vi "Async Logger.vi"(8 "error in":errorcluster, 11 "Logger Parameters":T1) -> (0 "error out":errorcluster, 3 "Logger Parameters":T1={"State"=enum."Initialize", "is Shutdown"=FALSE, "FIFO Refs"={"All System Channels Data"=refnum, "Status"=refnum, "CPU-RAM Data"=refnum}, "Buffers"={"Size"=0, "Current Index"=0, "Array Size"=0, "All System Channels Data"=[], "LOG Data"=[], "CPU-RAM Data"=[], "CPU-RAM Array"=[]}, "Log File"={"Path"=path "C:/logs/AdvancedTDMS_Telemetry_Prototype.tdms", "Ref"=refnum, "Overwrite File If Exists?"=FALSE, "System Channels"={"Names"=[], "Properties"=[], "Telemetry System Path"=""}}, "Target Info"={"Target Rate (Hz)"=0.0, "# of CPUs"=0, "TotalPhysMem (KB)"=0.0}, "Expected Channels"={"Names"=[], "Indexes"=[], "Count"=0}})   [LabVIEW 2019, in "Telemetry Engine.lvlib"]
uses:
  Telemetry Engine.lvlib
  Types/Logger Data.ctl
  Types/Async Logger State Data.ctl
  Types/System Channels.ctl
  Types/Target Info.ctl
  <vilib>/Platform/TimedLoop/XDataNode/timing_clust.ctl
  <vilib>/Platform/TimedLoop/XDataNode/nitl_modes.ctl
  <vilib>/Platform/TimedLoop/XDataNode/wakeup.ctl
  <vilib>/nisyscfg/Close (System).vi
  <vilib>/platform/TimedLoop/XDataNode/XDataNode.xnode
  <vilib>/Platform/TimedLoop/XDataNode/XDNodeRunTimeDep.lvlib
  <resource>/objmgr/nisysapi.rc
  <vilib>/nisyscfg/nisyscfg.lvlib
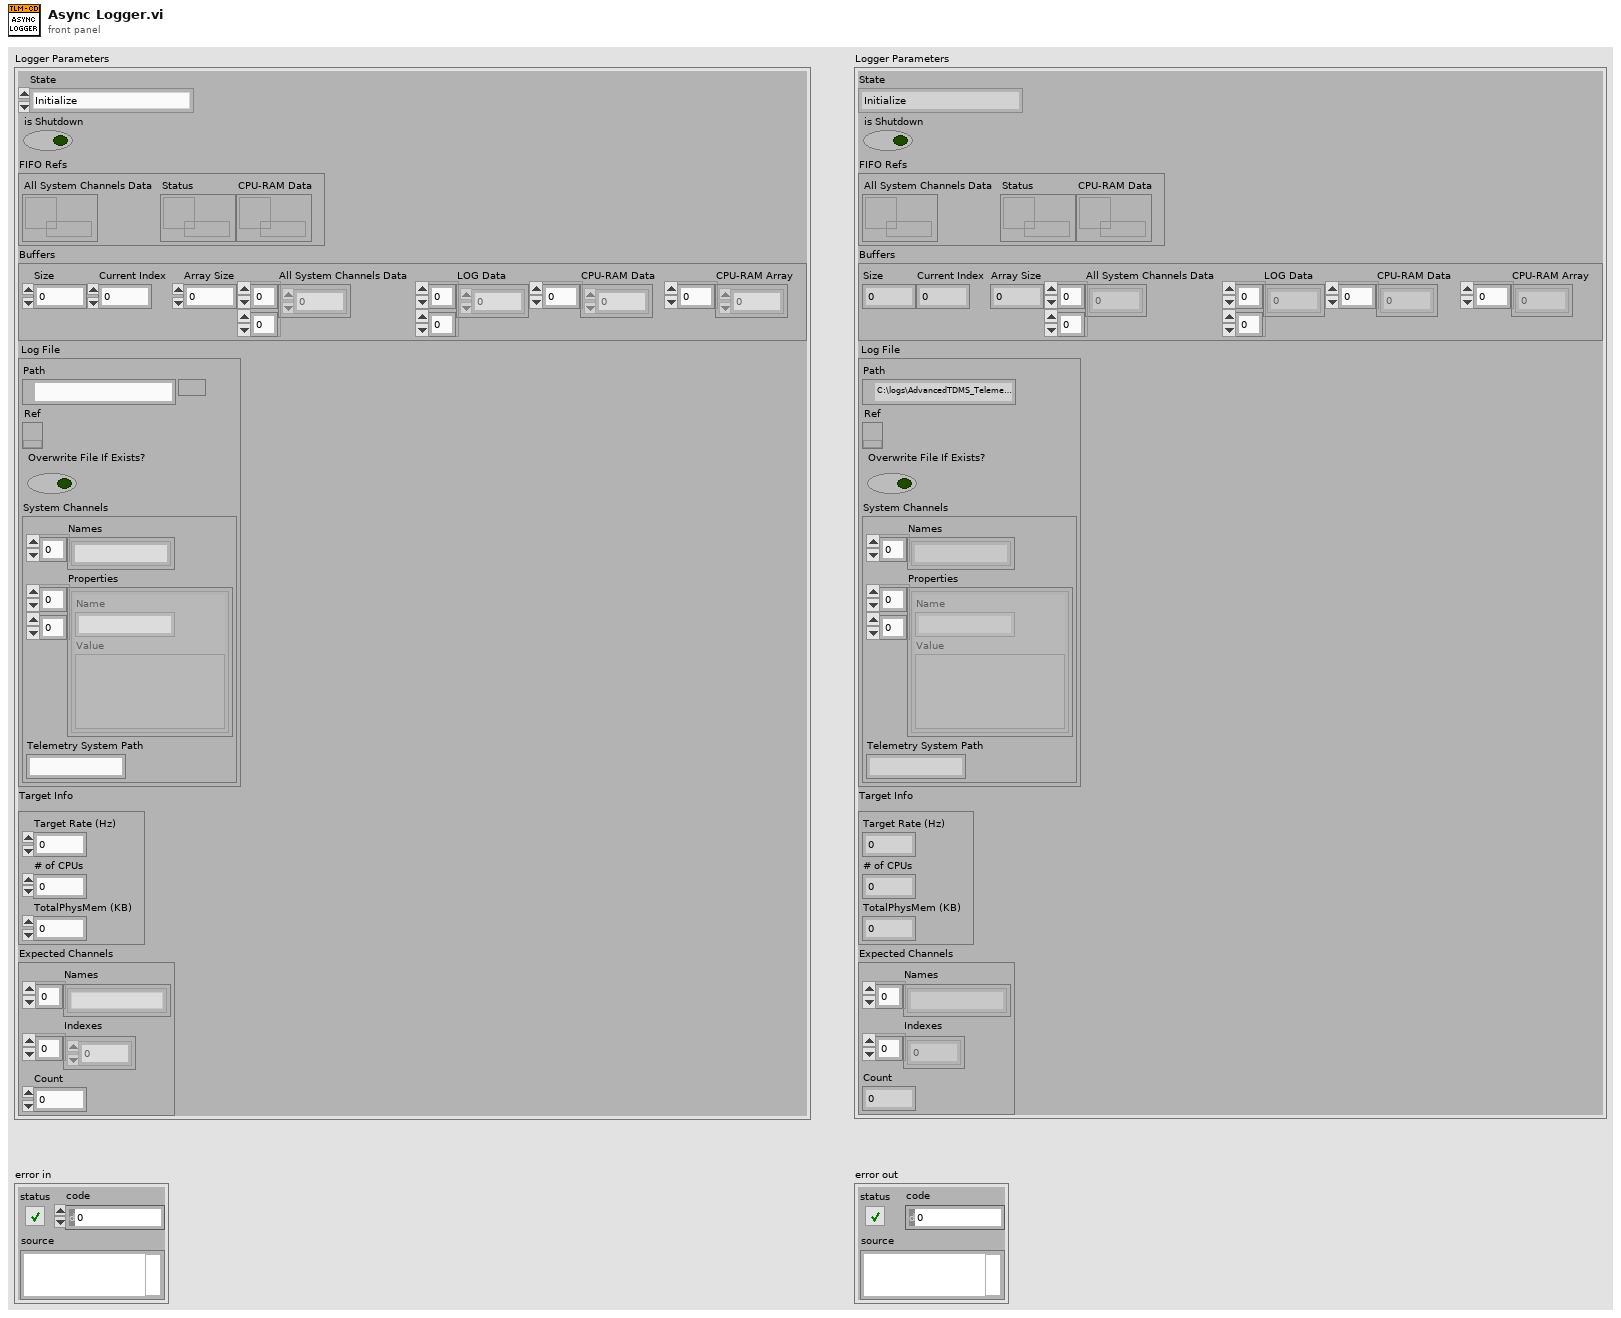
[diagram p1: front panel]
types:
  T1 = typedef "Telemetry Engine.lvlib/Logger Data.ctl" = cluster{"State":T2, "is Shutdown":bool, "FIFO Refs":cluster{"All System Channels Data":refnum<k33>, "Status":refnum<k33>, "CPU-RAM Data":refnum<k33>}, "Buffers":cluster{"Size":i32, "Current Index":i32, "Array Size":i32, "All System Channels Data":dbl[][], "LOG Data":dbl[][], "CPU-RAM Data":dbl[], "CPU-RAM Array":dbl[]}, "Log File":cluster{"Path":path, "Ref":refnum<k34>, "Overwrite File If Exists?":bool, "System Channels":T3}, "Target Info":T4, "Expected Channels":cluster{"Names":string[], "Indexes":i32[], "Count":i32}}
  T2 = typedef "Telemetry Engine.lvlib/Async Logger State Data.ctl" = enum16{"Initialize", "Read System Channels FIFO", "Filter System Channels", "Read CPU-RAM FIFO", "Log Data", "Shutdown"}
  T3 = typedef "Telemetry Engine.lvlib/System Channels.ctl" = cluster{"Names":string[], "Properties":cluster{"Name":string, "Value":variant}[][], "Telemetry System Path":string}
  T4 = typedef "Telemetry Engine.lvlib/Target Info.ctl" = cluster{"Target Rate (Hz)":dbl, "# of CPUs":u32, "TotalPhysMem (KB)":dbl}
  T5 = typedef "XDNodeRunTimeDep.lvlib/timing_clust.ctl" = cluster{"Expected End [f-1]":u64, "Actual End [f-1]":u64, "Finished Late? [f-1]":bool, "Expected End [i-1]":u64, "Actual End [i-1]":u64, "Finished Late? [i-1]":bool, "Expected Start [i]":u64, "Actual Start [i]":u64, "Expected Start [f]":u64, "Actual Start [f]":u64, "Source Name":string, "Structure Name":string, "Period":i64, "Deadline":i64, "Offset":i64, "Start":i64, "Priority":i32, "Timeout":i32, "Mode":T6, "Wakeup Reason":T7, "Error":errorcluster, "Source Type":string, "Secondary Source Type":string, "Global End Time":u64, "Global Start Time":u64, "Frame Duration":u64, "Iteration Duration":u64, "Assigned CPU":i32, "I/O Scan Engine Mode":u32}
  T6 = typedef "XDNodeRunTimeDep.lvlib/nitl_modes.ctl" = enum32{"No Change", "Process missed periods, maintain original phase", "Discard missed periods, maintain original phase", "Process missed periods, ignore original phase", "Discard missed periods, ignore original phase"}
  T7 = typedef "XDNodeRunTimeDep.lvlib/wakeup.ctl" = enum32{"Normal", "Aborted", "Asynchronous wakeup", "Timing source error", "Timed loop error", "Timeout"}
  T8 = typedef "NI_Real-Time Target Support.lvlib/RT CPU Load.ctl" = cluster{"Total (%)":dbl, "Time Critical (%)":dbl, "Timed Structures (%)":dbl, "High (%)":dbl, "Above Normal (%)":dbl, "Normal (%)":dbl, "Background (%)":dbl, "Idle (%)":dbl, "ISR (%)":dbl}
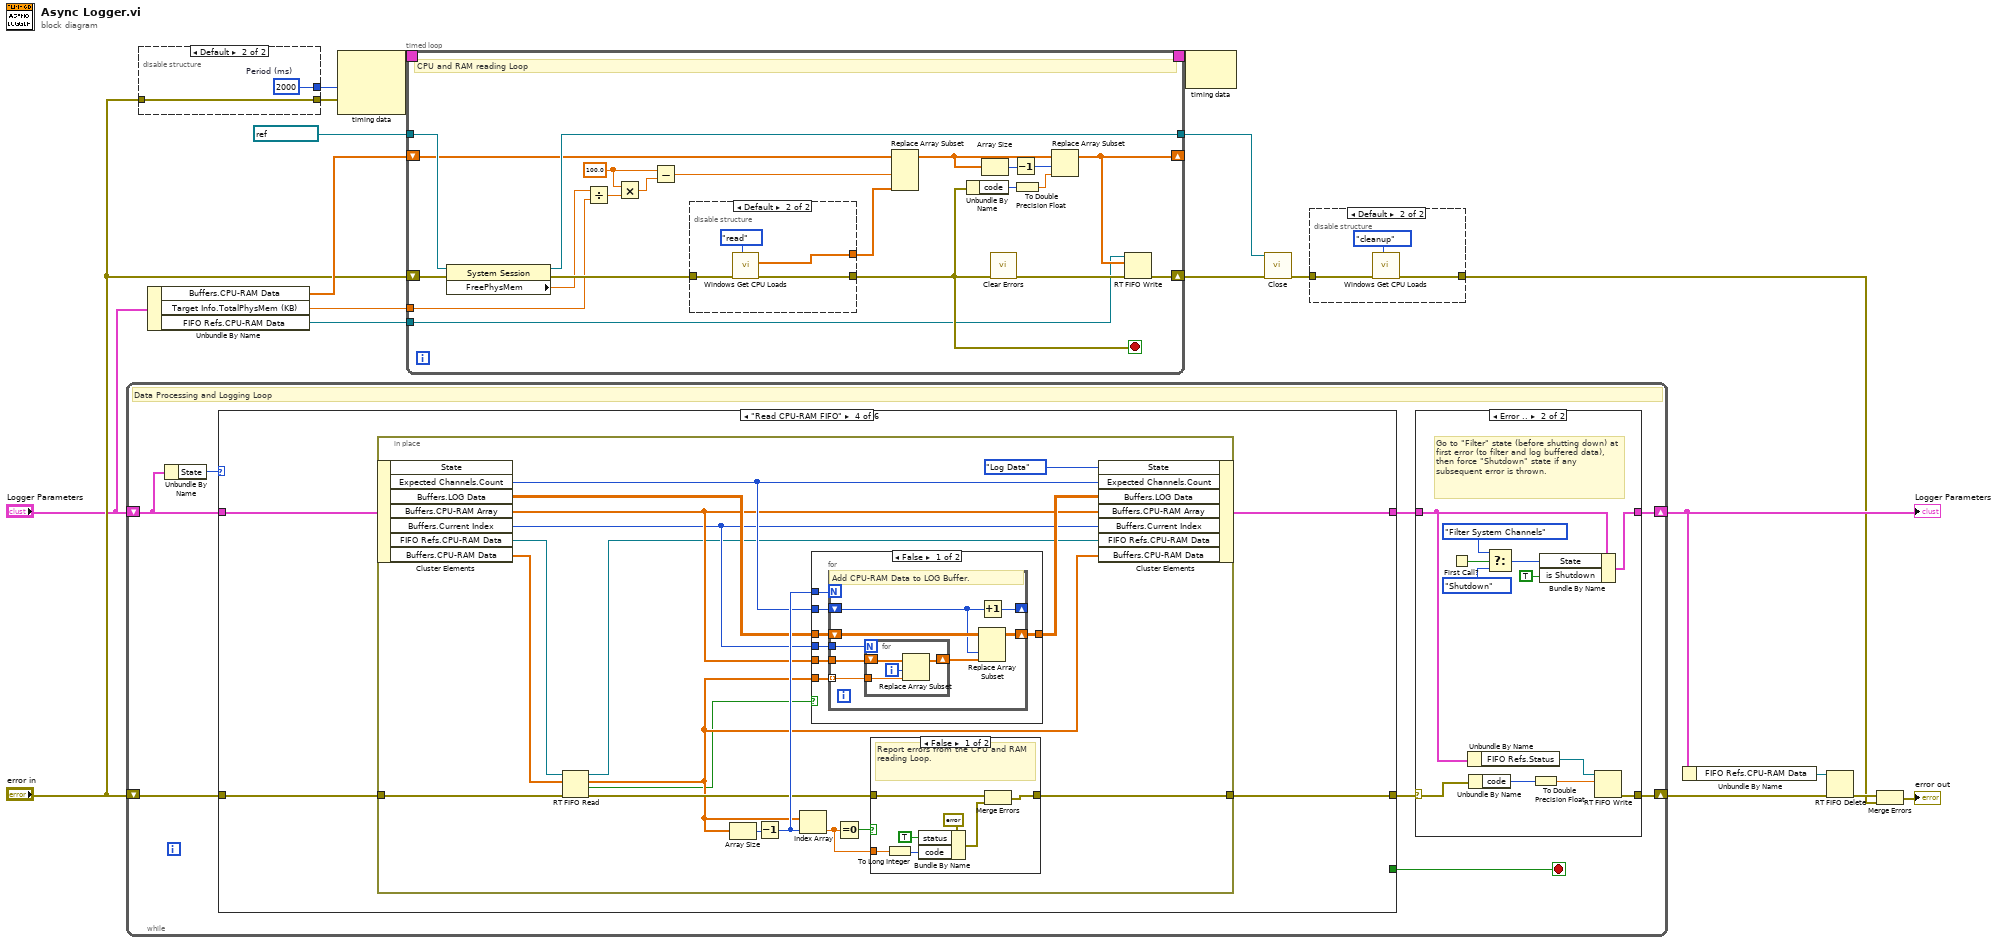
[diagram p0: block diagram]
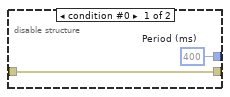
[diagram p3: hidden frame]
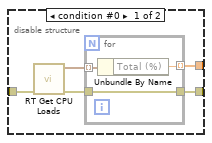
[diagram p4: hidden frame]
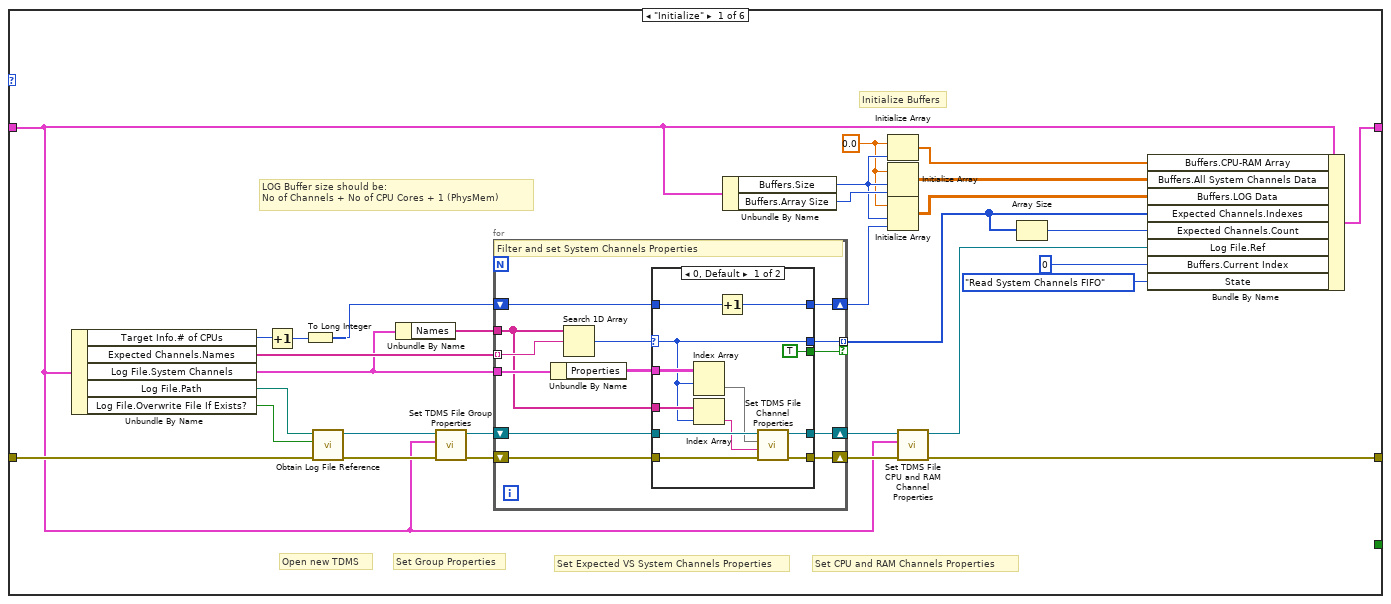
[diagram p5: hidden frame]
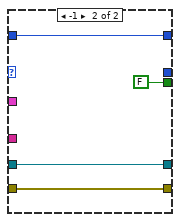
[diagram p6: hidden frame]
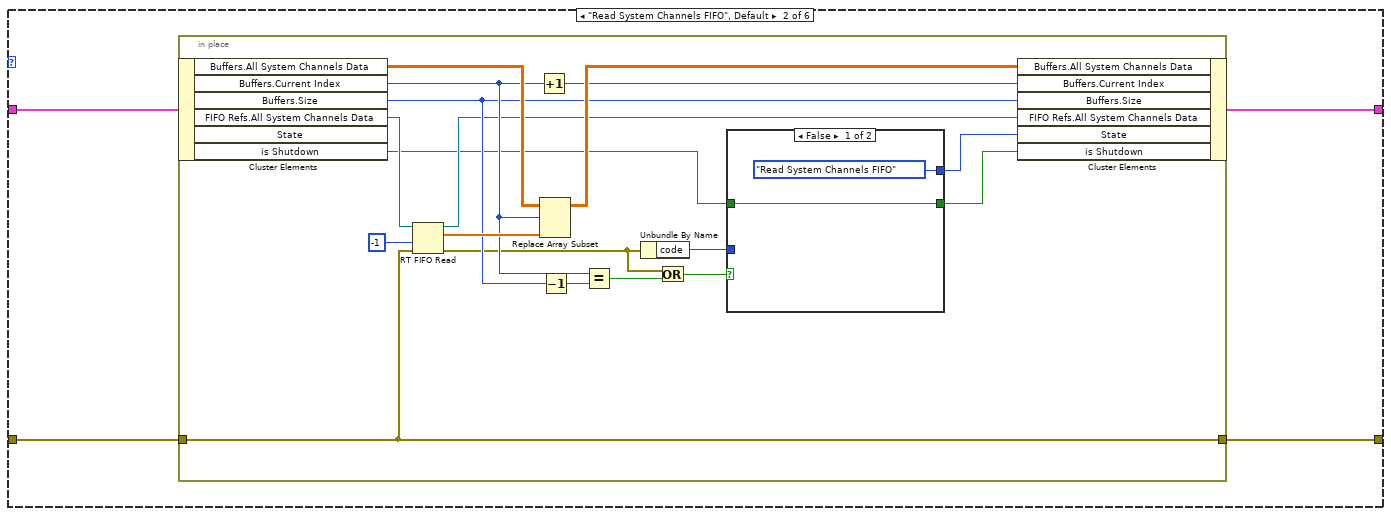
[diagram p7: hidden frame]
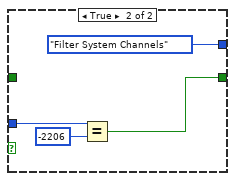
[diagram p8: hidden frame]
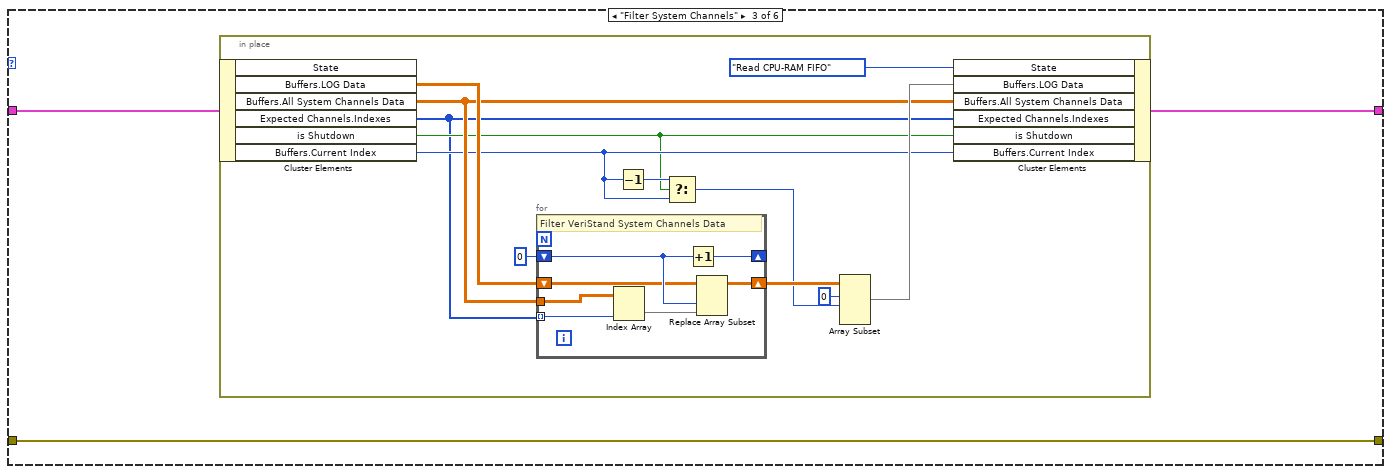
[diagram p9: hidden frame]
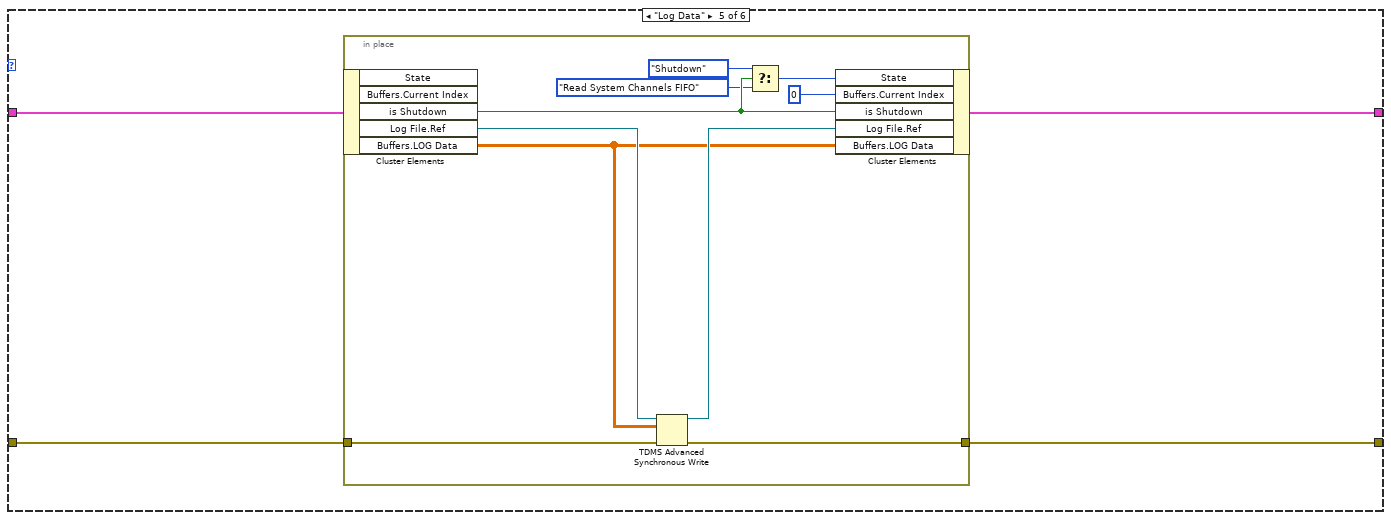
[diagram p12: hidden frame]
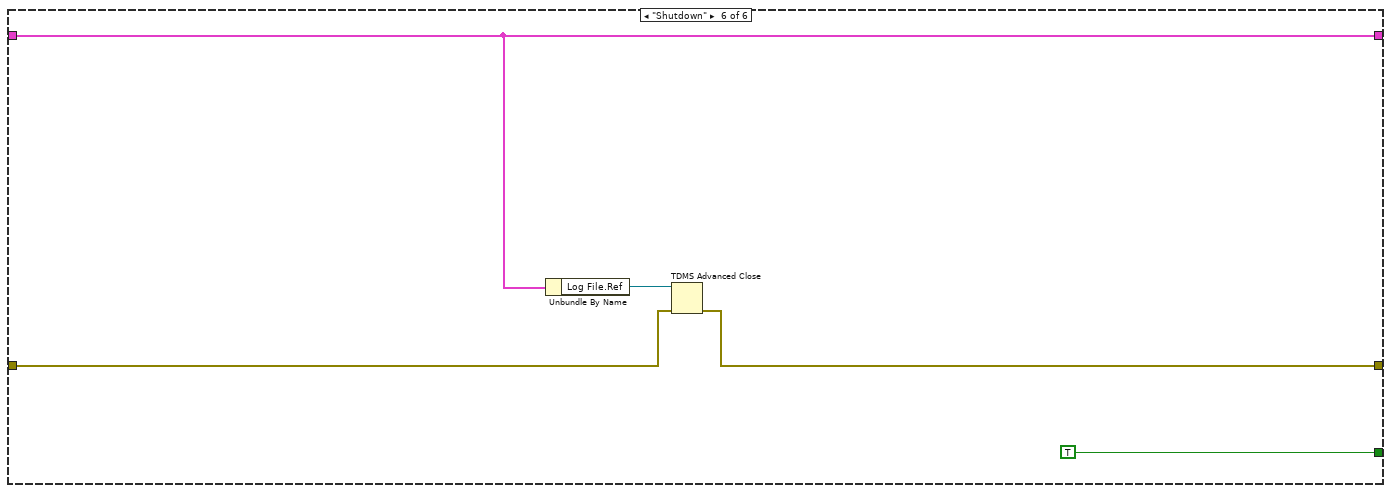
[diagram p13: hidden frame]
diagram:
  n1 = while {
    shift-right: [w22] -> w12
    shift-left: "Logger Parameters" -> [w21]
    shift-right: [w25] -> w14
    shift-left: "error in" -> [w26]
    stop <- w27 stop-if-true
    # "Data Processing and Logging Loop"
    n2 = Unbundle By Name(w21) -> ("State"=w20:T2)
    n3 = case shown="\"Read CPU-RAM FIFO\"" w20 {
      tunnel: [_ _ _ _ _ TRUE] -> w27
      tunnel: w21 -> [w28 w87 w117 w140 w188 w204]
      tunnel: [w55 w90 w116 w139 w187 w204] -> w23
      tunnel: [w37 w88 w115 w137 w189 w201] -> w24
      tunnel: w26 -> [w50 w89 w115 w138 w190 w202]
      frame "Initialize" {
        w29 = 0.0 ("element")
        # "Initialize Buffers"
        # "Set CPU and RAM Channels Properties"
        # "Set Expected VS System Channels Properties"
        # "Set Group Properties"
        # "Open new TDMS"
        # "LOG Buffer size should be:\nNo of Channels + No of CPU Cores + 1 (PhysMem)"
        n4 = Unbundle By Name(w28) -> ("Target Info.# of CPUs"=w41:u32, "Expected Channels.Names"=w47:string[], "Log File.System Channels"=w42:T3, "Log File.Path"=w49:path, "Log File.Overwrite File If Exists?"=w51:bool)
        n5 = Increment(x=w41) -> (x+1=w40:u32)
        n6 = To Long Integer(number=w40) -> (32bit integer=w39:i32)
        n7 = call "Obtain Log File Reference.vi"("error in"=w50, "Overwrite File If Exists?"=w51, "Log File Path"=w49) -> ("error out"=w45:errorcluster, "Log File Refnum out"=w43:refnum<k34>)  [unwired: 7 in]
        n8 = Unbundle By Name(w42) -> ("Names"=w48:string[])
        n9 = call "Set TDMS File Group Properties.vi"("error in (no error)"=w45, "Logger Parameters"=w28, "Refnum in"=w43) -> ("error out"=w46:errorcluster, "Refnum out"=w44:refnum<k34>)  [unwired: 7 in]
        n10 = for {
          shift-right: [w68] -> w36
          shift-left: w44 -> [w69]
          shift-right: [w67] -> w38
          shift-left: w46 -> [w70]
          shift-right: [w65] -> w54
          shift-left: w39 -> [w66]
          tunnel: w47 -> [w63] mode=indexing
          tunnel: w48 -> [w58]
          tunnel: [w62] -> w33 mode=indexing if=w59
          tunnel: w42 -> [w61]
          # "Filter and set System Channels Properties"
          n11 = Unbundle By Name(w61) -> ("Properties"=w60:cluster{"Name":string, "Value":variant}[][])
          n12 = Search 1D Array(1D array=w58, element=w63) -> (index of element=w64:i32)  [unwired: 1 in]
          n13 = case shown="0, Default" w64 {
            selector: w64 -> [w72 _]
            tunnel: [w82 w86] -> w68
            tunnel: [w81 w84] -> w67
            tunnel: w70 -> [w80 w84]
            tunnel: w69 -> [w79 w86]
            tunnel: w66 -> [w78 w85]
            tunnel: [w77 w85] -> w65
            tunnel: [w72 _] -> w62
            tunnel: w60 -> [w76 _]
            tunnel: [TRUE FALSE] -> w59
            tunnel: w58 -> [w73 _]
            frame 0, Default {
              n14 = Index Array(array=w76, index (row)=w72) -> (element=w75:cluster{"Name":string, "Value":variant}[])  [unwired: 1 in]
              n15 = Index Array(array=w73, index=w72) -> (element=w71:string)
              n16 = Increment(x=w78) -> (x+1=w77:i32)
              n17 = call "Set TDMS File Channel Properties.vi"("error in (no error)"=w80, "Channel Name"=w71, "Channel Properties"=w75, "tdms file in"=w79) -> ("error out"=w81:errorcluster, "tdms file out"=w82:refnum<k34>)  [unwired: 6 in]
            }
            frame -1 {
            }
          }
        }
        n18 = Unbundle By Name(w28) -> ("Buffers.Size"=w30:i32, "Buffers.Array Size"=w57:i32)
        n19 = Initialize Array(w29, w30) -> (w31:dbl[])
        n20 = Initialize Array(w29, w30, w57) -> (w56:dbl[][])
        n21 = Initialize Array(w29, w30, w54) -> (w53:dbl[][])
        n22 = call "Set TDMS File CPU and RAM Channel Properties.vi"("error in (no error)"=w38, "Logger Parameters"=w28, "Refnum in"=w36) -> ("error out"=w37:errorcluster, "Refnum out"=w35:refnum<k34>)  [unwired: 7 in]
        n23 = Array Size(array=w33) -> (size(s)=w32:i32)
        n24 = Bundle By Name(cluster=w28, "Buffers.CPU-RAM Array"=w31, "Buffers.All System Channels Data"=w56, "Buffers.LOG Data"=w53, "Expected Channels.Indexes"=w33, "Expected Channels.Count"=w32, "Log File.Ref"=w35, "Buffers.Current Index"=0 ("Buffer Index"), "State"=Async_Logger_State_Data."Read System Channels FIFO") -> (w55:T1)
      }
      frame "Read System Channels FIFO", Default {
        n25 = in-place {
          in-place-border: w89 -> [w101]
          in-place-border: [w101] -> w88
          n26 = in-place-cluster #1(w87) -> ("Buffers.All System Channels Data"=w105:dbl[][], "Buffers.Current Index"=w104:i32, "Buffers.Size"=w100:i32, "FIFO Refs.All System Channels Data"=w99:refnum<k33>, "is Shutdown"=w92:bool)  [unwired: 1 out]
          n27 = RT FIFO Read(0:w99, 2:-1 ("timeout in ms (0)"), 3:w101) -> (8:w94:refnum<k33>, 9:w106:dbl[], 11:w95:errorcluster)  [unwired: 1 in, 2 out]
          n28 = Increment(x=w104) -> (x+1=w102:i32)
          n29 = Replace Array Subset(array=w105, new element=w106, index (row)=w104) -> (w103:dbl[][])  [unwired: 1 in]
          n30 = Decrement(x=w100) -> (x-1=w107:i32)
          n31 = Equal?(x=w104, y=w107) -> (x = y?=w96:bool)
          n32 = Unbundle By Name(w95) -> ("code"=w97:i32)
          n33 = Or(x=w95, y=w96) -> (x .or. y?=w98:bool)
          n34 = case shown="False" w98 {
            tunnel: w97 -> [_ w113]
            tunnel: w92 -> [w110 _]
            tunnel: [w110 w112] -> w93
            tunnel: [Async_Logger_State_Data."Read System Channels FIFO" ("State") Async_Logger_State_Data."Filter System Channels" ("State")] -> w91
            frame False {
            }
            frame True {
              n35 = Equal?(x=w113, y=-2206) -> (x = y?=w112:bool)
            }
          }
          n36 = in-place-cluster #1("Buffers.All System Channels Data"=w103, "Buffers.Current Index"=w102, "Buffers.Size"=w100, "FIFO Refs.All System Channels Data"=w94, "State"=w91, "is Shutdown"=w93) -> (w90:T1)
        }
      }
      frame "Filter System Channels" {
        n37 = in-place {
          n38 = in-place-cluster #2(w117) -> ("Buffers.LOG Data"=w124:dbl[][], "Buffers.All System Channels Data"=w122:dbl[][], "Expected Channels.Indexes"=w119:i32[], "is Shutdown"=w120:bool, "Buffers.Current Index"=w121:i32)  [unwired: 1 out]
          n39 = for {
            tunnel: w122 -> [w136]
            shift-right: [w132] -> w128
            shift-left: w124 -> [w134]
            shift-right: [w133] -> _
            shift-left: 0 -> [w135]
            tunnel: w119 -> [w130] mode=indexing
            # "Filter VeriStand System Channels Data"
            n40 = Index Array(array=w136, index (col)=w130) -> (element=w131:dbl[])  [unwired: 1 in]
            n41 = Increment(x=w135) -> (x+1=w133:i32)
            n42 = Replace Array Subset(array=w134, new element=w131, index (col)=w135) -> (w132:dbl[][])  [unwired: 1 in]
          }
          n43 = Decrement(x=w121) -> (x-1=w127:i32)
          n44 = Select(t=w127, s=w120, f=w121) -> (s? t:f=w125:i32)
          n45 = Array Subset(array=w128, index (row)=0 ("index"), length (row)=w125) -> (w123:dbl[][])  [unwired: 2 in]
          n46 = in-place-cluster #2("State"=Async_Logger_State_Data."Read CPU-RAM FIFO", "Buffers.LOG Data"=w123, "Buffers.All System Channels Data"=w122, "Expected Channels.Indexes"=w119, "is Shutdown"=w120, "Buffers.Current Index"=w121) -> (w116:T1)
        }
      }
      frame "Read CPU-RAM FIFO" {
        n47 = in-place {
          in-place-border: w138 -> [w156]
          in-place-border: [w151] -> w137
          n48 = in-place-cluster #3(w140) -> ("Expected Channels.Count"=w148:i32, "Buffers.LOG Data"=w150:dbl[][], "Buffers.CPU-RAM Array"=w147:dbl[], "Buffers.Current Index"=w146:i32, "FIFO Refs.CPU-RAM Data"=w143:refnum<k33>, "Buffers.CPU-RAM Data"=w144:dbl[])  [unwired: 1 out]
          n49 = RT FIFO Read(0:w143, 1:w144, 3:w156) -> (8:w142:refnum<k33>, 9:w145:dbl[], 10:w141:bool, 11:w155:errorcluster)  [unwired: 1 in, 1 out]
          n50 = Array Size(array=w145) -> (size(s)=w154:i32)
          n51 = Decrement(x=w154) -> (x-1=w158:i32)
          n52 = Index Array(array=w145, index=w158) -> (element=w152:dbl)
          n53 = case shown="False" w141 {
            tunnel: w158 -> [w165 _]
            tunnel: w150 -> [w164 w178]
            tunnel: [w163 w178] -> w149
            tunnel: w148 -> [w162 _]
            tunnel: w147 -> [w161 _]
            tunnel: w146 -> [w160 _]
            tunnel: w145 -> [w159 _]
            frame False {
              n54 = for {
                N: w165 -> [_]
                shift-right: [w173] -> w163
                shift-left: w164 -> [w172]
                shift-right: [w171] -> _
                shift-left: w162 -> [w170]
                tunnel: w161 -> [w169]
                tunnel: w160 -> [w167]
                tunnel: w159 -> [w166] mode=indexing
                # "Add CPU-RAM Data to LOG Buffer."
                n55 = for {
                  N: w167 -> [_]
                  shift-right: [w176] -> w168
                  shift-left: w169 -> [w177]
                  tunnel: w166 -> [w174]
                  i -> [w175]
                  n56 = Replace Array Subset(array=w177, new element=w174, index=w175) -> (w176:dbl[])
                }
                n57 = Increment(x=w170) -> (x+1=w171:i32)
                n58 = Replace Array Subset(array=w172, new element=w168, index (col)=w170) -> (w173:dbl[][])  [unwired: 1 in]
              }
            }
            frame True {
              # "If CPU-RAM FIFO is empty use the previous values."
            }
          }
          n59 = Equal To 0?(x=w152) -> (x = 0?=w153:bool)
          n60 = case shown="False" w153 {
            tunnel: w152 -> [w185 _]
            tunnel: w155 -> [w180 w186]
            tunnel: [w179 w186] -> w151
            frame False {
              # "Report errors from the CPU and RAM reading Loop."
              n61 = To Long Integer(number=w185) -> (32bit integer=w183:i32)
              n62 = Bundle By Name(cluster=errorcluster {"status"=FALSE, "code"=0, "source"=""} ("error out"), "status"=TRUE, "code"=w183) -> (w181:errorcluster)
              n63 = Merge Errors(w180, w181) -> (w179:errorcluster)
            }
            frame True {
            }
          }
          n64 = in-place-cluster #3("State"=Async_Logger_State_Data."Log Data", "Expected Channels.Count"=w148, "Buffers.LOG Data"=w149, "Buffers.CPU-RAM Array"=w147, "Buffers.Current Index"=w146, "FIFO Refs.CPU-RAM Data"=w142, "Buffers.CPU-RAM Data"=w145) -> (w139:T1)
        }
      }
      frame "Log Data" {
        n65 = in-place {
          in-place-border: w190 -> [w200]
          in-place-border: [w199] -> w189
          n66 = in-place-cluster #4(w188) -> ("is Shutdown"=w195:bool, "Log File.Ref"=w198:refnum<k34>, "Buffers.LOG Data"=w191:dbl[][])  [unwired: 2 out]
          n67 = TDMS Advanced Synchronous Write(8:w200, 10:w191, 11:w198) -> (0:w199:errorcluster, 3:w194:refnum<k34>)
          n68 = Select(t=Async_Logger_State_Data."Shutdown" ("State"), s=w195, f=Async_Logger_State_Data."Read System Channels FIFO" ("State")) -> (s? t:f=w197:T2)
          n69 = in-place-cluster #4("State"=w197, "Buffers.Current Index"=0 ("Buffers.Index"), "is Shutdown"=w195, "Log File.Ref"=w194, "Buffers.LOG Data"=w191) -> (w187:T1)
        }
      }
      frame "Shutdown" {
        n70 = Unbundle By Name(w204) -> ("Log File.Ref"=w203:refnum<k34>)
        n71 = TDMS Advanced Close(8:w202, 11:w203) -> (0:w201:errorcluster)  [unwired: 2 in, 1 out]
      }
    }
    n72 = case shown="Error .." w24 {
      selector: w24 -> [w207 w217]
      tunnel: [w207 w212] -> w25
      tunnel: w23 -> [w206 w215]
      tunnel: [w206 w214] -> w22
      frame No Error {
      }
      frame Error {
        # "Go to \"Filter\" state (before shutting down) at first error (to filter and log buffered data), then force \"Shutdown\" state if any subsequent error is thrown."
        # "Go to Log state at first error (to empty log buffer), then to Shutdown if any subsequent error is thrown."
        n73 = First Call?() -> (First Call?: T/F=w211:bool)
        n74 = Unbundle By Name(w215) -> ("FIFO Refs.Status"=w218:refnum<k33>)
        n75 = Unbundle By Name(w217) -> ("code"=w216:i32)
        n76 = Select(t=Async_Logger_State_Data."Filter System Channels" ("State"), s=w211, f=Async_Logger_State_Data."Shutdown" ("State")) -> (s? t:f=w210:T2)
        n77 = To Double Precision Float(number=w216) -> (double precision float=w219:dbl)
        n78 = Bundle By Name(cluster=w215, "State"=w210, "is Shutdown"=TRUE) -> (w214:T1)
        n79 = RT FIFO Write(0:w218, 1:w219) -> (11:w212:errorcluster)  [unwired: 3 in, 3 out]
      }
    }
  }
  "Logger Parameters" <- w12
  n80 = disable-structure shown="Default" {
    disable-tunnel: [w221 w222] -> w1
    disable-tunnel: "error in" -> [w220 w223]
    disable-tunnel: [w220 w223] -> w10
    frame condition #0 {
      w221 = i64 400  # Period (ms)
    }
    frame condition #1 (active) {
      w222 = i64 2000  # Period (ms)
    }
  }
  n81 = Unbundle By Name("Logger Parameters") -> ("Buffers.CPU-RAM Data"=w5:dbl[], "Target Info.TotalPhysMem (KB)"=w7:dbl, "FIFO Refs.CPU-RAM Data"=w6:refnum<k33>)
  n82 = node-c288(w1, w10) -> (w19:T5)  [unwired: 1 in]
  n83 = timed-loop {
    timing: w19 -> [_]
    timing-out: [_] -> w18
    shift-right: [w236] -> _
    shift-left: w5 -> [w239]
    tunnel: w7 -> [w227]
    tunnel: refnum<k21> "localhost" ("System Session") -> [w245]
    tunnel: [w244] -> w16
    tunnel: w6 -> [w226]
    shift-right: [w225] -> w3
    shift-left: "error in" -> [w224]
    stop <- w229 stop-if-true
    w241 = 100.0 ("x")
    # "CPU and RAM reading Loop"
    n84 = property class="System Session"(reference=w245, error in=w224) -> (reference out=w244:refnum<k21>, error out=w237:errorcluster, "FreePhysMem"=w233:dbl)
    n85 = Divide(x=w233, y=w227) -> (x/y=w243:dbl)
    n86 = Multiply(x=w241, y=w243) -> (x*y=w242:dbl)
    n87 = Subtract(x=w241, y=w242) -> (x-y=w230:dbl)
    n88 = disable-structure shown="Default" {
      disable-tunnel: [w248 w256] -> w229
      disable-tunnel: w237 -> [w247 w257]
      disable-tunnel: [w246 w254] -> w231
      frame condition #0 {
        n89 = call <vilib>:"RT Get CPU Loads.vi"("error in (no error)"=w247) -> ("error out"=w249:errorcluster, "CPU loads"=w250:T8[])  [unwired: 9 in]
        n90 = for {
          tunnel: w250 -> [w253] mode=indexing
          tunnel: w249 -> [w252]
          tunnel: [w252] -> w248
          tunnel: [w251] -> w246 mode=indexing
          n91 = Unbundle By Name(w253) -> ("Total (%)"=w251:dbl)
        }
      }
      frame condition #1 (active) {
        n92 = call "Windows Get CPU Loads.vi"("Action"=enum16{"init", "read", "cleanup"}."read", "error in (no error)"=w257) -> ("error out"=w256:errorcluster, "CPU Loads"=w254:dbl[])  [unwired: 7 in, 1 out]
      }
    }
    n93 = Replace Array Subset(array=w239, new element #1=w230, new element #2=w231) -> (w232:dbl[])  [unwired: 2 in]
    n94 = Unbundle By Name(w229) -> ("code"=w240:i32)
    n95 = Array Size(array=w232) -> (size(s)=w238:i32)
    n96 = call <vilib>:"Clear Errors.vi"("error in (no error)"=w229) -> ("error out"=w228:errorcluster)  [unwired: 5 in, 1 out]
    n97 = Decrement(x=w238) -> (x-1=w235:i32)
    n98 = To Double Precision Float(number=w240) -> (double precision float=w234:dbl)
    n99 = Replace Array Subset(array=w232, new element=w234, index=w235) -> (w236:dbl[])
    n100 = RT FIFO Write(0:w226, 1:w236, 3:w228) -> (11:w225:errorcluster)  [unwired: 2 in, 3 out]
  }
  n101 = node-c288(w18) -> ()  [unwired: 1 out]
  n102 = call-poly <vilib>:"Close.vi"("error in (no error)"=w3, "Session in"=w16) -> ("error out"=w9:errorcluster)  [unwired: 9 in]
  n103 = disable-structure shown="Default" {
    disable-tunnel: w9 -> [w260 w262]
    disable-tunnel: [w260 w261] -> w8
    frame condition #0 {
    }
    frame condition #1 (active) {
      n104 = call "Windows Get CPU Loads.vi"("Action"=enum16{"init", "read", "cleanup"}."cleanup", "error in (no error)"=w262) -> ("error out"=w261:errorcluster)  [unwired: 7 in, 2 out]
    }
  }
  n105 = Unbundle By Name(w12) -> ("FIFO Refs.CPU-RAM Data"=w11:refnum<k33>)
  n106 = RT FIFO Delete(0:w11, 3:w14) -> (11:w13:errorcluster)  [unwired: 1 in]
  n107 = Merge Errors(w13, w8) -> (→"error out":errorcluster)
